vi "CmdConsole.Write to StdIn.vi"(8 "error in (no error)":errorcluster, 9 "Mult Lines":string[](array[string]), 10 "StdIn":string, 11 "CmdConsole in":refnum<class "CmdConsole.lvclass">) -> (0 "error out":errorcluster, 3 "CmdConsole out":refnum<class "CmdConsole.lvclass">)   [LabVIEW 2018, in "CmdConsole.lvclass"]
uses:
  CmdConsole.lvclass
  CmdConsole.lvclass/CmdConsole.ctl
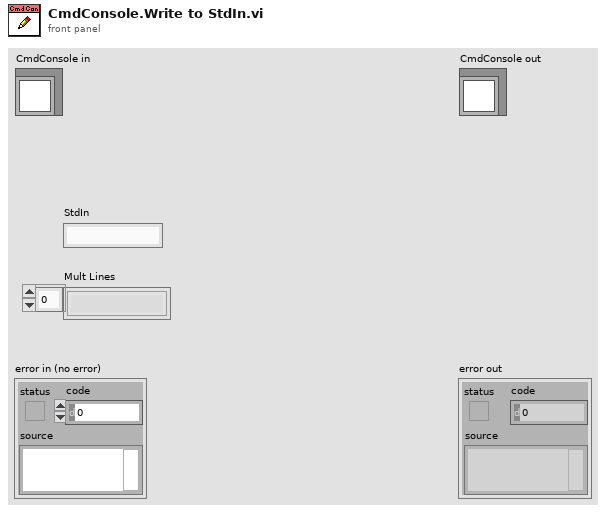
[diagram p1: front panel]
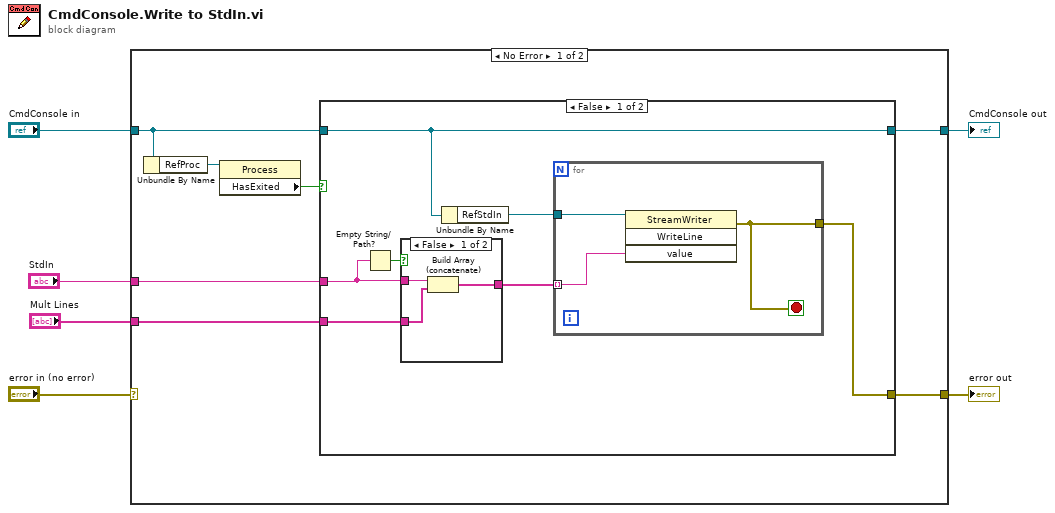
[diagram p0: block diagram]
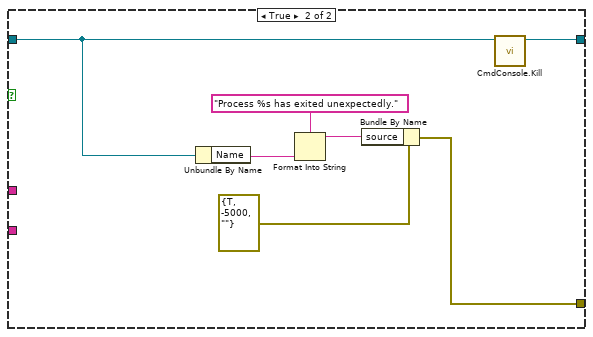
[diagram p3: hidden frame]
diagram:
  n1 = case shown="No Error" "error in (no error)" {
    selector: "error in (no error)" -> [_ w36]
    tunnel: [w11 w36] -> w5
    tunnel: [w10 w35] -> w3
    tunnel: "CmdConsole in" -> [w9 w35]
    tunnel: "Mult Lines" -> [w12 _]
    tunnel: "StdIn" -> [w13 _]
    frame No Error {
      n2 = Unbundle By Name(w9) -> ("RefProc"=w8:refnum<k24>)
      n3 = property class="Process"(reference=w8) -> ("HasExited"=w7:bool)  [unwired: 1 in, 2 out]
      n4 = case shown="False" w7 {
        tunnel: w9 -> [w14 w29]
        tunnel: w13 -> [w18 _]
        tunnel: w12 -> [w17 _]
        tunnel: [w15 w30] -> w11
        tunnel: [w14 w28] -> w10
        frame False {
          n5 = Empty String/Path?(string/path=w18) -> (empty?=w19:bool)
          n6 = case shown="False" w19 {
            tunnel: w18 -> [w23 _]
            tunnel: w17 -> [w22 w24]
            tunnel: [w21 w24] -> w16
            frame False {
              n7 = Build Array (concatenate)(w23, w22) -> (w21:string[])
            }
            frame True {
            }
          }
          n8 = Unbundle By Name(w14) -> ("RefStdIn"=w20:refnum<k24>)
          n9 = for {
            tunnel: w20 -> [w27]
            tunnel: w16 -> [w26] mode=indexing
            tunnel: [w25] -> w15
            stop <- w25 stop-if-true
            n10 = invoke class="StreamWriter" method="WriteLine"(reference=w27, "value"=w26) -> (error out=w25:errorcluster)  [unwired: 2 in, 3 out]
          }
        }
        frame True {
          n11 = Unbundle By Name(w29) -> ("Name"=w33:string)
          n12 = Format Into String(format string="Process %s has exited unexpectedly." ("source"), w33) -> (resulting string=w34:string)  [unwired: 2 in, 1 out]
          n13 = Bundle By Name(cluster=errorcluster {"status"=TRUE, "code"=-5000, "source"=""} ("error constant"), "source"=w34) -> (w30:errorcluster)
          n14 = call "CmdConsole.Kill.vi"("CmdConsole in"=w29) -> ("CmdConsole out"=w28:refnum<class "CmdConsole.lvclass">)  [unwired: 9 in, 1 out]
        }
      }
    }
    frame Error {
    }
  }
  "error out" <- w5
  "CmdConsole out" <- w3
